vi "simx Create Dummy.vi"(6 "operationMode":i32, 7 "objectHandle":i32, 8 "error in (no error)":errorcluster, 9 "colors":string, 10 "size":sgl, 11 "clientID":i32) -> (0 "error out":errorcluster, 3 "function return":i32, 5 "objectHandle out":i32)   [LabVIEW 2019, in "PXL_V-REP.lvlib"]
doc: "EXTAPI_DLLEXPORT simxInt simxCreateDummy(simxInt clientID,simxFloat size,const simxUChar* colors,simxInt* objectHandle,simxInt operationMode);"
uses:
  PXL_V-REP.lvlib
  <userlib>/V-REP/remoteApi.dll
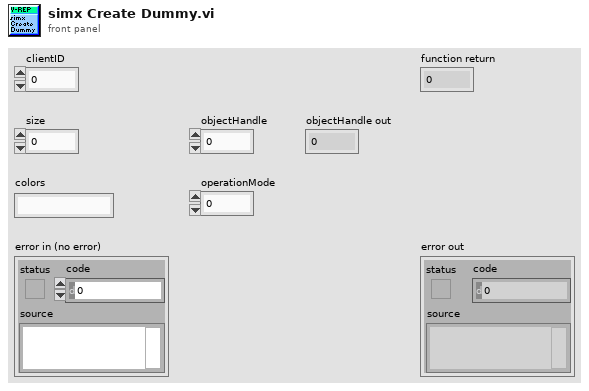
[diagram p1: front panel]
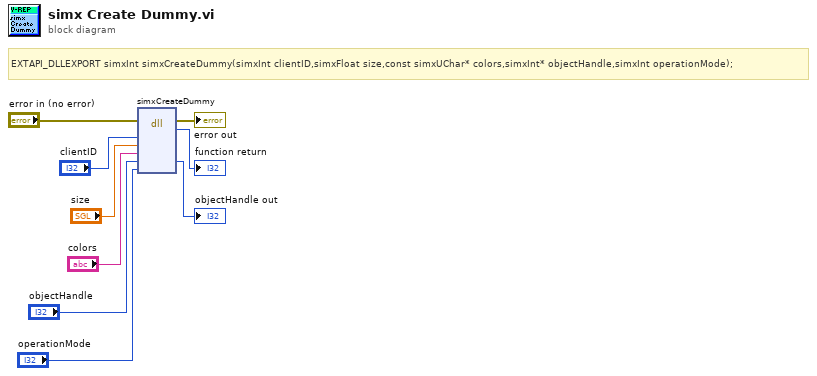
[diagram p0: block diagram]
diagram:
  # "EXTAPI_DLLEXPORT simxInt simxCreateDummy(simxInt clientID,simxFloat size,const simxUChar* colors,simxInt* objectHandle,simxInt operationMode);"
  n1 = dll-call lib="C:/Program Files (x86)/National Instruments/LabVIEW 2019/user.lib/V-REP/remoteApi.*" fn="simxCreateDummy"(error in="error in (no error)", "clientID"="clientID", "size"="size", "colors"="colors", "objectHandle"="objectHandle", "operationMode"="operationMode") -> (error out=→"error out":errorcluster, →"function return":i32, "objectHandle"=→"objectHandle out":i32)  [unwired: 6 in, 1 out]
